vi "CamTest.vi"() -> ()   [LabVIEW 2017]
uses:
  <vilib>/userdefined/High Color/IMAQdx.ctl
  <vilib>/vision/driver/NI_Vision_Acquisition_Software.lvlib
panel:
  in  "stop":bool
  out "Image":T1(plugin-control)
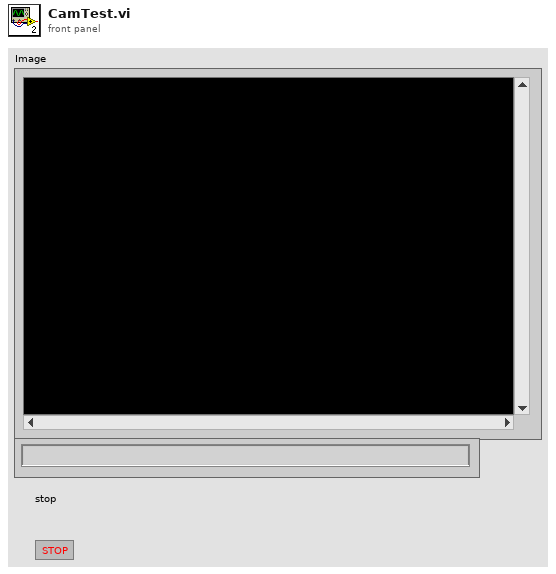
[diagram p1: front panel]
types:
  T1 = typedef "IMAQ Image.ctl" = refnum<image>
  T2 = typedef "IMAQdx.ctl" = refnum<k21>
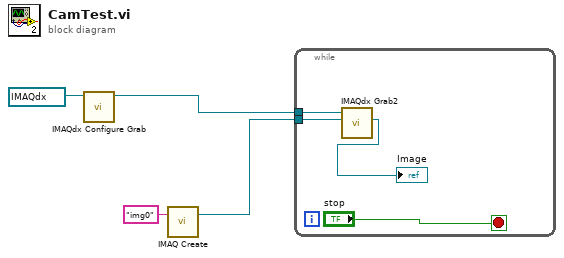
[diagram p0: block diagram]
diagram:
  n1 = call <vilib>:"IMAQdx Configure Grab.vi"("Session In"=T2 "cam2") -> ("Session Out"=w1:T2)  [unwired: 9 in, 1 out]
  n2 = call "IMAQ Create"("Image Name"="img0") -> ("New Image"=w3:T1)  [unwired: 4 in, 1 out]
  n3 = while {
    tunnel: w1 -> [w8]
    tunnel: w3 -> [w5]
    stop <- "stop" stop-if-true
    n4 = call <vilib>:"IMAQdx Grab2.vi"("Image In"=w5, "Session In"=w8) -> ("Image Out"=→"Image":T1)  [unwired: 6 in, 3 out]
  }
